vi "风扇温度正则表达式.vi"(10 "字符串":string, 11 "匹配之后":string) -> (3 "temp":string[](array[string]))   [LabVIEW 2015]
uses:
  <vilib>/regexp/Match Regular Expression.xnode
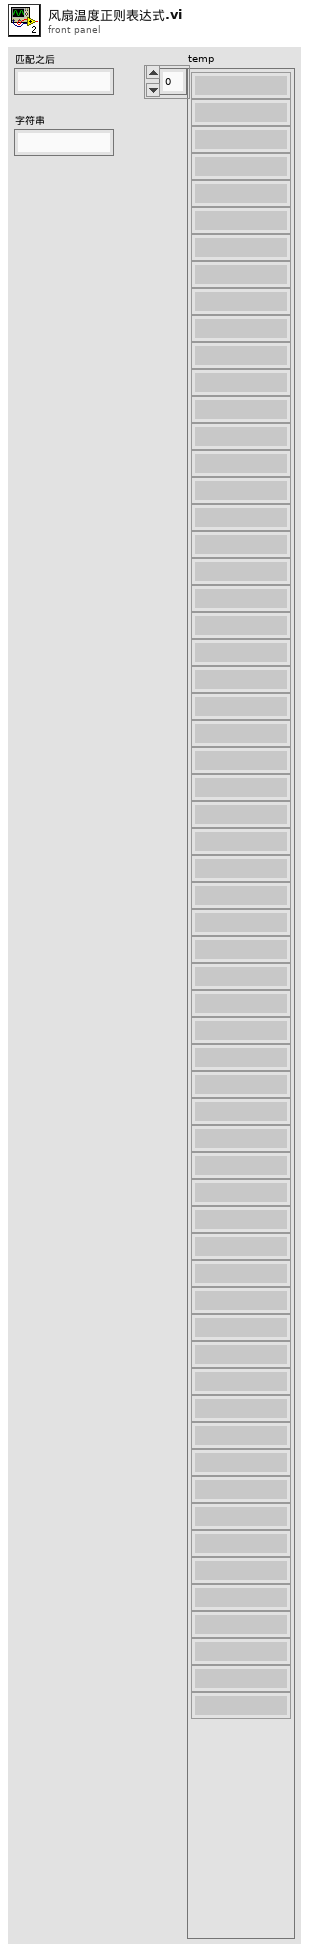
[diagram p1: front panel]
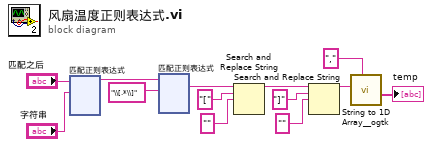
[diagram p0: block diagram]
diagram:
  n1 = xnode "匹配正则表达式"("输入字符串"="匹配之后", "正则表达式"="字符串") -> ("匹配之前"=w3:string)  [unwired: 4 in, 4 out]
  n2 = xnode "匹配正则表达式"("输入字符串"=w3, "正则表达式"="\\[.*\\]") -> ("所有匹配"=w5:string)  [unwired: 4 in, 4 out]
  n3 = Search and Replace String(input string=w5, search string="[" ("搜索字符串"), replace string="" ("替换字符串(\"\")")) -> (result string=w8:string)  [unwired: 5 in, 3 out]
  n4 = Search and Replace String(input string=w8, search string="]" ("搜索字符串"), replace string="" ("替换字符串(\"\")")) -> (result string=w11:string)  [unwired: 5 in, 3 out]
  n5 = call <userlib>:"String to 1D Array__ogtk.vi"("delimiter (Tab)"=",", "string"=w11) -> ("Array of Strings"=→"temp":string[])  [unwired: 9 in]
